vi "Queue_Macro.vi"(8 "error in":errorcluster, 9 "lithography_Offsets":cluster{"X":dbl, "Y":dbl}, 10 "Lithography Data In":T1(array[cluster]), 11 "Application":refnum<k7>) -> (0 "error out":errorcluster)   [LabVIEW 2016]
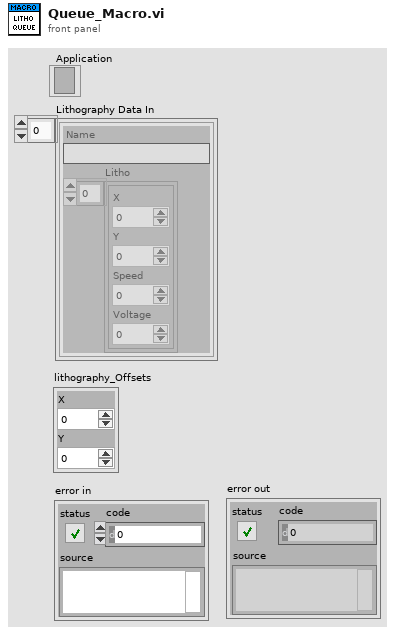
[diagram p1: front panel]
types:
  T1 = cluster{"Name":string, "Litho":cluster{"X":dbl, "Y":dbl, "Speed":dbl, "Voltage":dbl}[]}[]
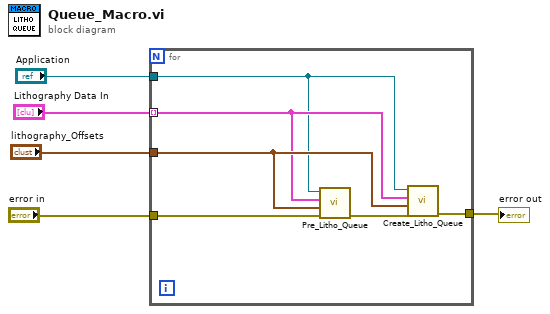
[diagram p0: block diagram]
diagram:
  n1 = for {
    tunnel: "Lithography Data In" -> [w8] mode=indexing
    tunnel: "Application" -> [w7]
    tunnel: "lithography_Offsets" -> [w9]
    tunnel: "error in" -> [w11]
    tunnel: [w6] -> w1
    n2 = call "Pre_Litho_Queue.vi"("error in"=w11, "lithography_Offsets"=w9, "Pattern Data"=w8, "Application"=w7) -> ("error out"=w10:errorcluster)  [unwired: 7 in]
    n3 = call "Create_Litho_Queue.vi"("error in"=w10, "lithography_Offsets"=w9, "Pattern Data"=w8, "Application"=w7) -> ("error out"=w6:errorcluster)  [unwired: 7 in]
  }
  "error out" <- w1
